vi "Localized Strings.vi"() -> ()   [LabVIEW 2020, in "Message Rescripter.lvlib"]
uses:
  Message Rescripter.lvlib
panel:
  in  "Select the reference method":string="Select the reference method:"
  in  "Rescript Message":string="Rescript Message"
  in  "Actor Framework":string="Actor Framework"
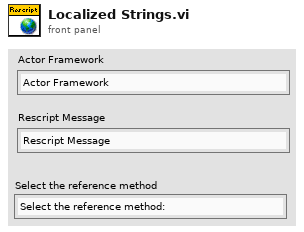
[diagram p1: front panel]
diagram:
